vi "Pcre2Compile8.vi"(8 "error in":errorcluster, 9 "pCompileContext":u64 format="%.0x", 10 "Options":u32 format="%.0x", 11 "Pattern":string) -> (0 "error out":errorcluster, 3 "pCode":u64 format="%.0x")   [LabVIEW 2021, in "libpcre2-8.lvlib"]
uses:
  libpcre2-8.lvlib
  libpcre2-8-x32.dll
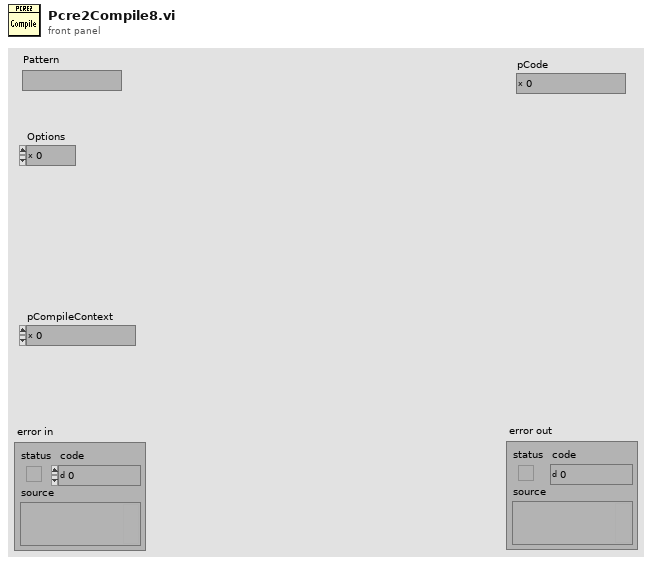
[diagram p1: front panel]
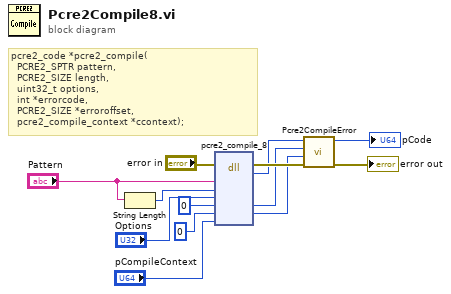
[diagram p0: block diagram]
diagram:
  # "pcre2_code *pcre2_compile(\n  PCRE2_SPTR pattern,\n  PCRE2_SIZE length, \n  uint32_t options, \n  int *errorcode, \n  PCRE2_SIZE *erroroffset, \n  pcre2_compile_context *ccontext);"
  n1 = String Length(string="Pattern") -> (length=w2:i32)
  n2 = dll-call lib="libpcre2-8-x*.dll" fn="pcre2_compile_8"(error in="error in", "pattern"="Pattern", "length"=w2, "options"="Options", "errorcode"=0, "erroroffset"=u64 0, "ctx"="pCompileContext") -> (error out=w8:errorcluster, "code"=w6:u64, "errorcode"=w4:i32, "erroroffset"=w3:u64)  [unwired: 6 in, 1 out]
  n3 = call "Pcre2CompileError.vi"("error in"=w8, "ErrorOffset"=w3, "ErrorCode"=w4, "pCode"=w6) -> ("error out"=→"error out":errorcluster, "pCode"=→"pCode":u64)  [unwired: 6 in]
